vi "Get MAC Address.vi"(8 "Error In":errorcluster) -> (0 "Error Out":errorcluster, 3 "MAC address":string)   [LabVIEW 2021, in "Utilities.lvlib"]
uses:
  Utilities.lvlib
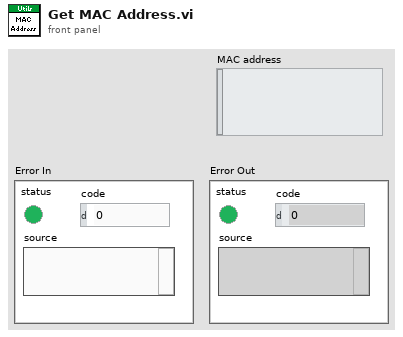
[diagram p1: front panel]
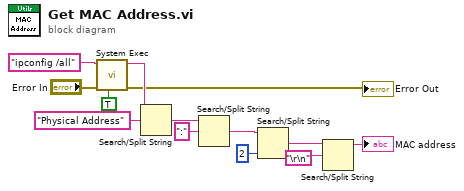
[diagram p0: block diagram]
diagram:
  n1 = call <vilib>:"System Exec.vi"("run minimized? (F)"=TRUE, "error in (no error)"="Error In", "command line"="ipconfig /all") -> ("error out"=→"Error Out":errorcluster, "standard output"=w11:string)  [unwired: 5 in, 2 out]
  n2 = Search/Split String(string=w11, search string/char (-)="Physical Address") -> (match + rest of string=w9:string)  [unwired: 1 in, 2 out]
  n3 = Search/Split String(string=w9, search string/char (-)=":") -> (match + rest of string=w5:string)  [unwired: 1 in, 2 out]
  n4 = Search/Split String(string=w5, offset (0)=2) -> (match + rest of string=w4:string)  [unwired: 1 in, 2 out]
  n5 = Search/Split String(string=w4, search string/char (-)="\r\n") -> (substring before match=→"MAC address":string)  [unwired: 1 in, 2 out]
